vi "Check_SN.vi"(8 "error in (no error)":errorcluster caption="错误输入（无错误）", 10 "输入sn":string[](array[string]), 11 "测试SN 2":refnum<vi>) -> (0 "error out":errorcluster caption="错误输出", 2 "检查结果":bool[](array[boolean]), 3 "测试SN 3":refnum<vi>)   [LabVIEW 2018]
uses:
  <vilib>/Utility/miscctls.llb/LVRowAndColumnTypeDef.ctl
panel:
  out "输出数组":string[][](array[string])
  in  "测试SN":i32(listbox)
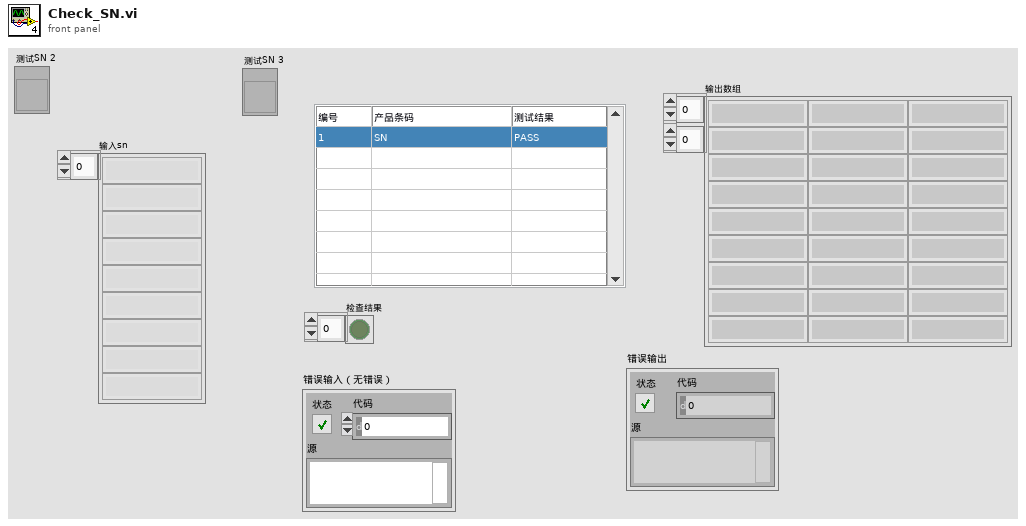
[diagram p1: front panel]
types:
  T1 = typedef "LVRowAndColumnTypeDef.ctl" = cluster{"Row":i32, "Column":i32}
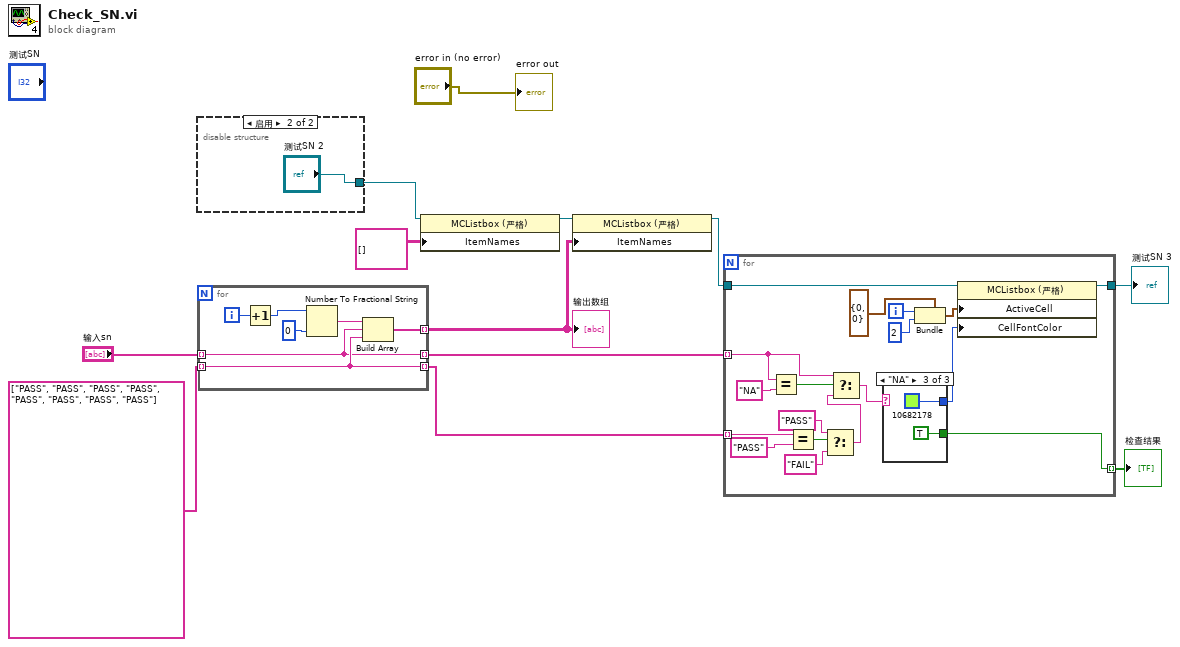
[diagram p0: block diagram]
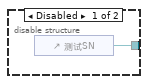
[diagram p2: hidden frame]
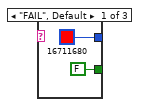
[diagram p3: hidden frame]
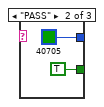
[diagram p4: hidden frame]
diagram:
  n1 = disable-structure shown="启用" {
    disable-tunnel: [w13 "测试SN 2"] -> w9
    frame Disabled {
      n2 = control-ref of="测试SN"() -> (w13:refnum<vi>)
    }
    frame Enabled {
    }
  }
  n3 = for {
    tunnel: [w18] -> w12 mode=indexing
    tunnel: "输入sn" -> [w15] mode=indexing
    tunnel: string[] ["PASS", "PASS", "PASS", "PASS", "PASS", "PASS", "PASS", "PASS"] -> [w16] mode=indexing
    tunnel: [w16] -> w2 mode=indexing
    tunnel: [w15] -> w1 mode=indexing
    i -> [w20]
    n4 = Increment(x=w20) -> (x+1=w17:i32)
    n5 = Number To Fractional String(number=w17, precision (6)=i16 0 ("精度(6)")) -> (F-format string=w19:string)  [unwired: 2 in]
    n6 = Build Array(w19, w15, w16) -> (w18:string[])
  }
  "输出数组" <- w12
  n7 = property class="MCListbox (严格)"(reference=w9, "ItemNames"=string[][] []) -> (reference out=w11:refnum<vi>)  [unwired: 1 in, 1 out]
  n8 = property class="MCListbox (严格)"(reference=w11, "ItemNames"=w12) -> (reference out=w8:refnum<vi>)  [unwired: 1 in, 1 out]
  n9 = for {
    tunnel: w8 -> [w39]
    tunnel: w2 -> [w33] mode=indexing
    tunnel: [w31] -> w6
    tunnel: [w30] -> w4 mode=indexing
    tunnel: w1 -> [w27] mode=indexing
    i -> [w37]
    n10 = Equal?(x=w27, y="NA") -> (x = y?=w28:bool)
    n11 = Equal?(x=w33, y="PASS") -> (x = y?=w26:bool)
    n12 = Select(t="PASS" ("y"), s=w26, f="FAIL" ("y")) -> (s? t:f=w23:string)
    n13 = Select(t=w27, s=w28, f=w23) -> (s? t:f=w22:string)
    n14 = case shown="\"NA\"" w22 {
      tunnel: [u32 16711680 u32 40705 u32 10682178] -> w35
      tunnel: [FALSE TRUE TRUE] -> w30
      frame "FAIL", Default {
      }
      frame "PASS" {
      }
      frame "NA" {
      }
    }
    n15 = Bundle(cluster=T1 {"Row"=0, "Column"=0} ("活动单元格:活动单元格"), "Row"=w37, "Column"=2) -> (w36:T1)
    n16 = property class="MCListbox (严格)"(reference=w39, "ActiveCell"=w36, "CellFontColor"=w35) -> (reference out=w31:refnum<vi>)  [unwired: 1 in, 1 out]
  }
  "测试SN 3" <- w6
  "检查结果" <- w4
  "error out" <- "error in (no error)"
